vi "OscGetWCM_max-Com-Exec.vi"(6 "Timeout (10000 ms)":u32=10000, 8 "error in (no error)":errorcluster, 11 "Oscilloscope in":refnum<class "Oscilloscope.lvclass">) -> (0 "error out":errorcluster, 3 "Oscilloscope out":refnum<class "Oscilloscope.lvclass">)   [LabVIEW 2015, in "Oscilloscope.lvclass"]
uses:
  Oscilloscope.lvclass
  GeneralFunctionality/GeneralFunctionality.lvclass/GeneralFunctionality.ctl
  Oscilloscope.lvclass/Oscilloscope.ctl
  dependecies/ControlsVIs/Clusters-def/Standard Command.ctl
  dependecies/ControlsVIs/Clusters-def/OSc-WCM_max_value.ctl
  Config/Config.lvclass
  TELEDINE_LECROY/LeCroy Wave Series/LeCroy Wave Series.lvlib
  GeneralFunctionality/GeneralFunctionality.lvclass
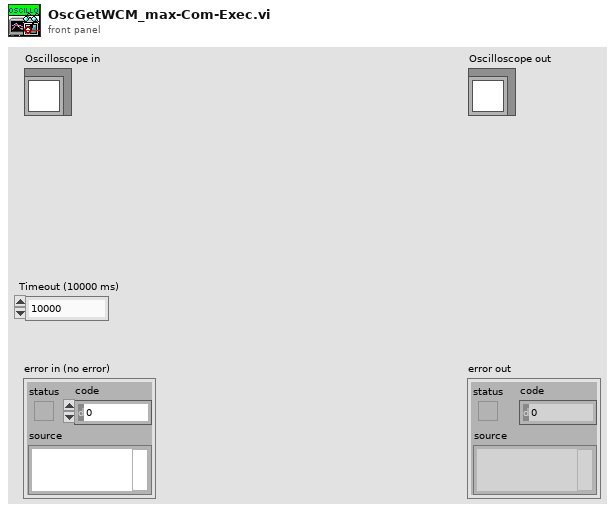
[diagram p1: front panel]
types:
  T1 = typedef "Oscilloscope.lvclass/OSc-WCM_max_value.ctl" = cluster{"WCM_max_value":dbl}
  T2 = typedef "Standard Command.ctl" = cluster{"command":string, "data":variant}
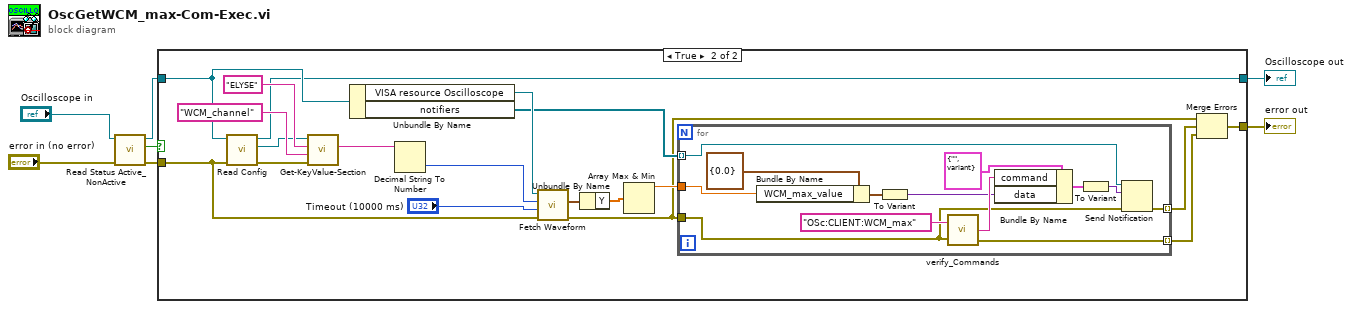
[diagram p0: block diagram]
diagram:
  n1 = call "Read Status Active_NonActive.vi"("error in (no error)"="error in (no error)", "GeneralFunctionality in"="Oscilloscope in") -> ("error out"=w1:errorcluster, "Status Active/NonActive"=w2:bool, "GeneralFunctionality out"=w3:refnum<class "Oscilloscope.lvclass">)  [unwired: 7 in]
  n2 = case shown="True" w2 {
    tunnel: [w9 w20] -> w7
    tunnel: [w8 w10] -> w6
    tunnel: w3 -> [w9 w26]
    tunnel: w1 -> [w8 w25]
    frame False {
    }
    frame True {
      n3 = call "Read Config.vi"("error in (no error)"=w25, "GeneralFunctionality en entrée"=w26) -> ("error out"=w24:errorcluster, "Config.lvclass"=w21:refnum<class "Config.lvclass">, "GeneralFunctionality en sortie"=w20:refnum<class "Oscilloscope.lvclass">)  [unwired: 7 in]
      n4 = call-dynamic "Get-KeyValue-Section.vi"("error in (no error)"=w24, "Key"="WCM_channel", "Section"="ELYSE", "Config in"=w21) -> ("Value"=w19:string)  [unwired: 5 in, 2 out]
      n5 = Unbundle By Name(w26) -> ("VISA resource Oscilloscope"=w28:refnum<visa-resource-name>, "notifiers"=w15:refnum<notifier>[])
      n6 = Decimal String To Number(string=w19) -> (number=w18:i32)  [unwired: 2 in, 1 out]
      n7 = call "Fetch Waveform.vi"("error in (no error)"=w25, "Timeout (10000 ms)"="Timeout (10000 ms)", "Source (0: Channel 1)"=w18, "VISA resource name"=w28) -> ("error out"=w13:errorcluster, "Waveform Graph"=w17:waveform(dbl))  [unwired: 5 in, 1 out]
      n8 = Unbundle By Name(w17) -> ("Y"=w16:dbl[])
      n9 = Array Max & Min(array=w16) -> (max value=w14:dbl)  [unwired: 3 out]
      n10 = for {
        tunnel: w15 -> [w35] mode=indexing
        tunnel: [w36] -> w11 mode=indexing
        tunnel: [w32] -> w12 mode=indexing
        tunnel: w14 -> [w31]
        tunnel: w13 -> [w30]
        n11 = Bundle By Name(cluster=T1 {"WCM_max_value"=0.0} ("ELYSE pulses counter"), "WCM_max_value"=w31) -> (w38:T1)
        n12 = To Variant(anything=w38) -> (Variant=w39:variant)
        n13 = call "verify_Commands.vi"("Command"="OSc:CLIENT:WCM_max" ("command"), "error in"=w30) -> ("Command out"=w41:string, "error out"=w36:errorcluster)  [unwired: 1 out]
        n14 = Bundle By Name(cluster=T2 {"command"="", "data"=variant} ("command"), "command"=w41, "data"=w39) -> (w34:T2)
        n15 = To Variant(anything=w34) -> (Variant=w33:variant)
        n16 = Send Notification(notification=w33, notifier=w35, error in (no error)=w30) -> (error out=w32:errorcluster)  [unwired: 1 out]
      }
      n17 = Merge Errors(w13, w12, w11) -> (w10:errorcluster)
    }
  }
  "error out" <- w6
  "Oscilloscope out" <- w7
